vi "Main.vi"(8 "error in (no error)":errorcluster) -> ()   [LabVIEW 2014, in "PmuImpairModule.lvlib"]
uses:
  PmuImpairModule.lvlib
  <userlib>/NIST/ModuleAdminLib/ModuleAdmin/ModuleAdmin.lvclass
  PublicAPI/Arguments/Requests/clStopArgument.ctl
  PmuImpairPlugins/PmuImpairPluginBase_class/PmuImpairPluginBase.lvclass
  <userlib>/NIST/ModuleAdminLib/ModuleAdmin/ModuleAdmin.lvclass/ModuleAdmin.ctl
  <userlib>/NIST/BaseClasses/BasePlugin_class/BasePlugin.lvclass/BasePlugin.ctl
  PmuImpairPlugins/PmuImpairPluginBase_class/TypeDefs/clImpairConfig.ctl
  PmuImpairPlugins/PmuImpairPluginBase_class/PmuImpairPluginBase.lvclass/PmuImpairPluginBase.ctl
  PublicAPI/Arguments/Requests/dblImpairParams.ctl
  EventPlugins/EventPluginBaseClass/TypeDefs/clEvtReportArray.ctl
  EventPlugins/EventPluginBaseClass/TypeDefs/clEvtReport.ctl
  EventPlugins/EventPluginBaseClass/TypeDefs/dblEvtSignalArray.ctl
  EventPlugins/EventPluginBaseClass/TypeDefs/clEvtConfig.ctl
  <vilib>/Utility/error.llb/DialogType.ctl
  <userlib>/NIST/ModuleAdminLib/ModuleAdmin/Accessors/Read ShowPanel_.vi
  <userlib>/NIST/ModuleAdminLib/ModuleAdmin/Accessors/Write ShowPanel_.vi
  <userlib>/NIST/BaseClasses/BasePlugin_class/Accessors/Write PluginIniFilePath.vi
  <userlib>/NIST/BaseClasses/BasePlugin_class/Accessors/Read PluginIniFilePath.vi
  PmuImpairPlugins/PmuImpairPluginBase_class/Accessors/Write BusNumber.vi
  PmuImpairPlugins/PmuImpairPluginBase_class/Accessors/Read BusNumber.vi
  PmuImpairPlugins/PmuImpairPluginBase_class/Accessors/Write dblEventSignalArray.vi
  PmuImpairPlugins/PmuImpairPluginBase_class/Accessors/Write dblEventParams.vi
  PmuImpairPlugins/PmuImpairPluginBase_class/Accessors/Write clEvtConfig.vi
  <userlib>/NIST/ModuleAdminLib/ModuleAdmin/Accessors/Read CloneRegRef.vi
  <vilib>/Utility/error.llb/Error Cluster From Error Code.vi
  PmuImpairPlugins/PmuImpairPluginBase_class/Accessors/Write clImpairConfig.vi
  PmuImpairPlugins/PmuImpairPluginBase_class/Accessors/Read clImpairConfig.vi
  PmuImpairPlugins/PmuImpairPluginBase_class/Accessors/Write dblImpairParams.vi
  PmuImpairPlugins/PmuImpairPluginBase_class/Accessors/Read dblImpairParams.vi
  PmuImpairPlugins/PmuImpairPluginBase_class/Accessors/Get ImpairReports.vi
  <vilib>/ErrorRing/Error Ring.xnode
  <userlib>/NIST/ModuleAdminLib/CloneRegistration/CloneRegistration.lvclass
  <userlib>/NIST/ModuleAdminLib/ModuleAdmin.lvlib
  <userlib>/NIST/BaseClasses/Object_class/BaseObject.lvclass
  EventPlugins/EventPluginBaseClass/EventPluginBaseClass.lvclass
panel:
  out "error out":errorcluster
  in  "ModuleAdmin":refnum<class "ModuleAdmin.lvclass">
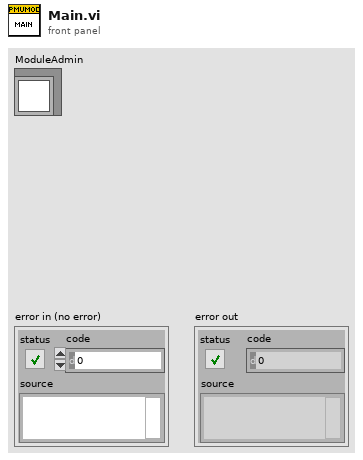
[diagram p1: front panel]
types:
  T1 = typedef "PmuImpairModule.lvlib/clRequestEvents.ctl" = cluster{"StopRequest":refnum<user-event>, "LoadPluginRequest":refnum<user-event>, "WriteImpairConfig":refnum<user-event>, "ReadImpairConfig":refnum<user-event>, "WriteImpairParams":refnum<user-event>, "ReadImpairParams":refnum<user-event>, "WriteEvtReports":refnum<user-event>, "GetImpairReports":refnum<user-event>, "ReadPathToPluginRequest":refnum<user-event>, "WriteEvtSignal":refnum<user-event>, "WriteEvtConfig":refnum<user-event>, "WriteEvtParams":refnum<user-event>, "ReadBusNumber":refnum<user-event>, "WriteBusNumber":refnum<user-event>, "ShowPanel":refnum<user-event>}
  T2 = typedef "PmuImpairModule.lvlib/clBroadcastEvents.ctl" = cluster{"DidInit":refnum<user-event>, "StatusUpdate":refnum<user-event>, "ErrorReport":refnum<user-event>, "DidStop":refnum<user-event>, "ImpairConfig":refnum<user-event>, "ImpairParams":refnum<user-event>, "ImpairReports":refnum<user-event>, "PathToPlugin":refnum<user-event>, "BusNumber":refnum<user-event>}
  T3 = typedef "PmuImpairModule.lvlib/clStopArgument.ctl" = cluster{"Exit via Stop Module Req?":bool, "Wait for Module to stop?":bool, "ModuleAdmin":refnum<class "ModuleAdmin.lvclass">}
  T4 = enum32{"Invalid", "Standard", "Closed", "Hidden", "Minimized", "Maximized"}
  T5 = typedef "PmuImpairPlugins.lvlib/PmuImpairPluginBase.lvclass/clImpairConfig.ctl" = cluster{"FilterType":string, "bPosSeq":bool}
  T6 = typedef "PmuImpairModule.lvlib/dblImpairParams.ctl" = dbl[][]
  T7 = typedef "EventPlugins.lvlib/EventPluginBaseClass.lvclass/clEvtReportArray.ctl" = T8[]
  T8 = typedef "EventPlugins.lvlib/EventPluginBaseClass.lvclass/clEvtReport.ctl" = cluster{"Timestamp":dbl, "Synx":cdb[], "Freq":dbl, "ROCOF":dbl, "ID":i16}
  T9 = typedef "EventPlugins.lvlib/EventPluginBaseClass.lvclass/dblEvtSignalArray.ctl" = dbl[][]
  T10 = typedef "EventPlugins.lvlib/EventPluginBaseClass.lvclass/clEvtConfig.ctl" = cluster{"T0(UTC)":dbl, "F0":dbl, "Fs":i32, "FSamp":u32, "bPosSeq":bool}
  T11 = typedef "DialogType.ctl" = u16
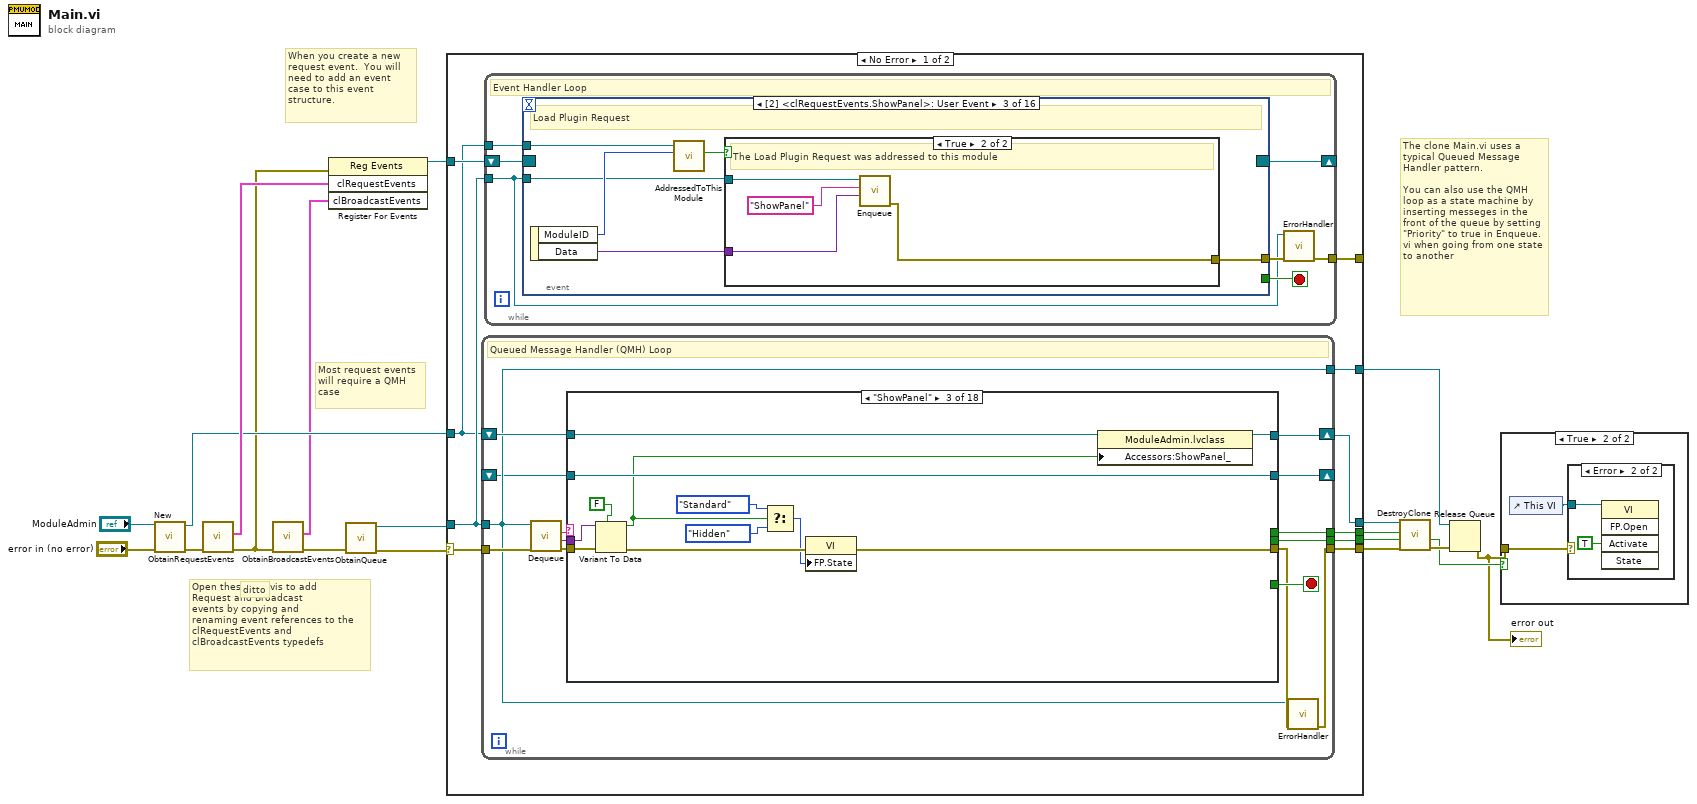
[diagram p0: block diagram]
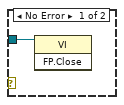
[diagram p3: hidden frame]
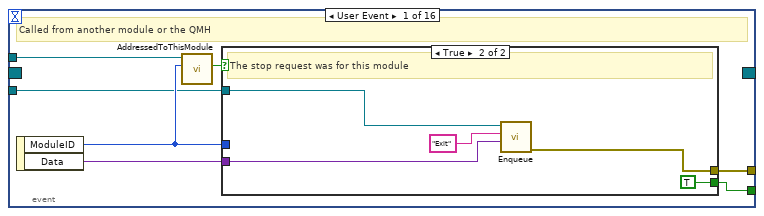
[diagram p4: hidden frame]
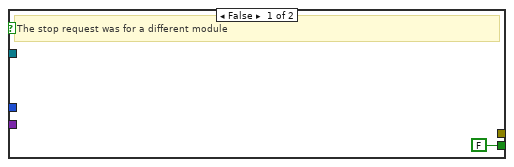
[diagram p5: hidden frame]
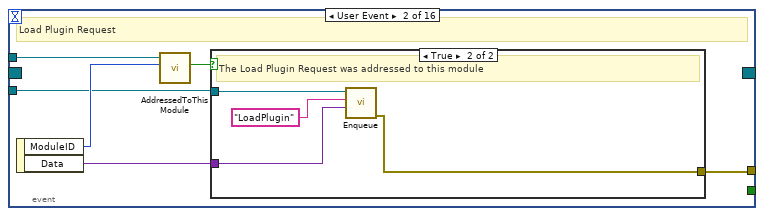
[diagram p6: hidden frame]
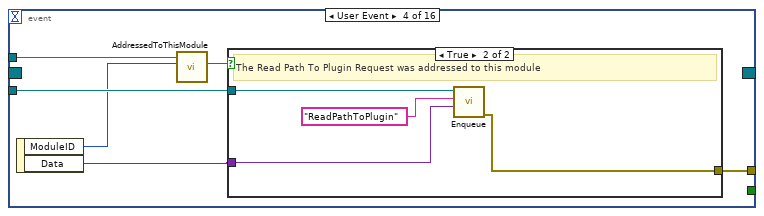
[diagram p9: hidden frame]
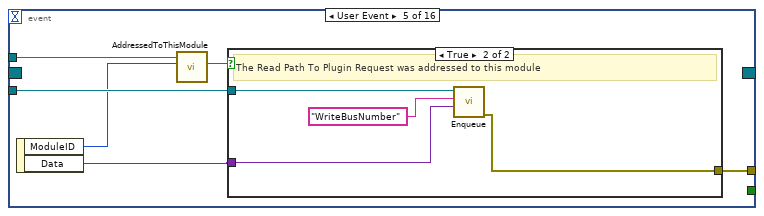
[diagram p11: hidden frame]
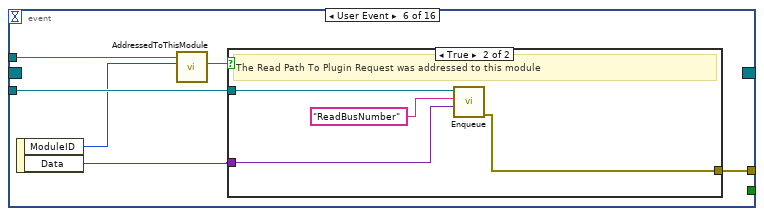
[diagram p13: hidden frame]
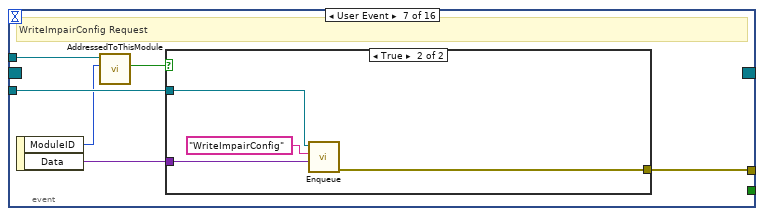
[diagram p15: hidden frame]
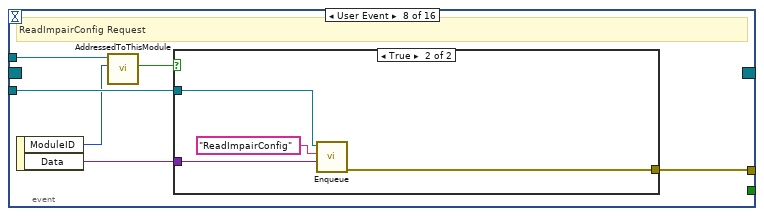
[diagram p17: hidden frame]
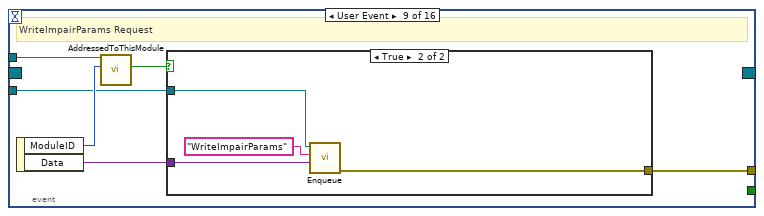
[diagram p19: hidden frame]
diagram:
  # "The clone Main.vi uses a typical Queued Message Handler pattern.  \n\nYou can also use the QMH loop as a state machine by inserting messeges in the front of the queue by setting \"Priority\" to true in Enqueue.vi when going from one state to another"
  # "Open these two vis to add\nRequest and Broadcast \nevents by copying and \nrenaming event references to the \nclRequestEvents and \nclBroadcastEvents typedefs"
  # "ditto"
  # "Most request events\nwill require a QMH\ncase"
  # "When you create a new request event.  You will need to add an event case to this event structure."
  n1 = call <userlib>:"New.vi"("error in (no error)"="error in (no error)", "ModuleAdmin"="ModuleAdmin") -> ("error out"=w17:errorcluster, "ModuleAdmin"=w13:refnum<class "ModuleAdmin.lvclass">)  [unwired: 7 in, 1 out]
  n2 = call "ObtainRequestEvents.vi"("error in (no error)"=w17) -> ("error out"=w10:errorcluster, "clRequestEvents"=w16:T1)  [unwired: 9 in]
  n3 = call "ObtainBroadcastEvents.vi"("error in (no error)"=w10) -> ("error out"=w11:errorcluster, "clBroadcastEvents"=w9:T2)  [unwired: 9 in]
  n4 = register-events(error in=w10, w16, w9) -> (reference out=w8:refnum<event-registration>)  [unwired: 1 in, 1 out]
  n5 = call "ObtainQueue.vi"("error in (no error)"=w11) -> ("error out"=w15:errorcluster, "MessageQueue"=w14:refnum<queue>)  [unwired: 9 in]
  n6 = case shown="No Error" w15 {
    selector: w15 -> [w29 w500]
    tunnel: w14 -> [w27 w496]
    tunnel: w13 -> [w24 w497]
    tunnel: [w28 w498] -> w7
    tunnel: [w26 w496] -> w12
    tunnel: w8 -> [w25 _]
    tunnel: [w23 w495] -> w5
    tunnel: [w22 _] -> w4
    tunnel: [w21 _] -> w3
    tunnel: [w20 _] -> _
    frame No Error {
      n7 = while {
        tunnel: w27 -> [w206]
        tunnel: w29 -> [w215]
        tunnel: [w208] -> w28
        tunnel: [w206] -> w26
        tunnel: [w210] -> w22
        tunnel: [w209] -> w21
        shift-right: [w205] -> _
        shift-left: _ -> [w204]
        shift-right: [w203] -> w23
        shift-left: w24 -> [w211]
        stop <- w216 stop-if-true
        # "Queued Message Handler (QMH) Loop"
        n8 = call "Dequeue.vi"("error in (no error)"=w215, "MessageQueue"=w206) -> ("error out"=w214:errorcluster, "Message Data"=w212:variant, "Message"=w213:string)  [unwired: 6 in, 1 out]
        n9 = case shown="\"ShowPanel\"" w213 {
          selector: w213 -> [w221 _ _ _ _ _ _ _ _ _ _ _ _ _ _ _ _ _]
          tunnel: [_ _ _ _ _ _ _ _ _ _ _ _ _ _ _ _ TRUE _] -> w216
          tunnel: w211 -> [w224 w253 w265 w281 w323 w337 w351 w364 w375 w384 w397 w403 w416 w429 w442 w463 w465 w486]
          tunnel: [w220 w242 w267 w280 w321 w336 w350 w357 w366 w385 w392 w407 w420 w433 w446 w455 w472 w477] -> w207
          tunnel: w214 -> [_ _ w273 w283 w325 w339 w352 w362 w373 w383 w398 w405 w418 w431 w444 w457 w471 w485]
          tunnel: w212 -> [_ _ w272 w284 _ w340 w353 _ _ w382 _ w406 w419 w432 w445 _ w470 w484]
          tunnel: [_ _ _ _ _ _ _ _ _ _ _ _ _ _ _ _ w468 _] -> w210
          tunnel: [_ _ _ _ _ _ _ _ _ _ _ _ _ _ _ _ w467 _] -> w209
          tunnel: [w218 refnum<class "PmuImpairPluginBase.lvclass"> refnum ("PmuImpairPlugins.lvlib:PmuImpairPluginBase.lvclass") w266 w276 w322 w331 w345 w360 w371 w379 w394 w401 w414 w427 w440 w462 w466 w476] -> w205
          tunnel: w204 -> [w218 _ w266 w282 w324 w332 w346 w363 w374 w380 w399 w402 w415 w428 w441 w460 w466 w476]
          tunnel: [w217 w233 w263 w274 w319 w328 w341 w354 w365 w376 w389 w400 w413 w426 w439 w452 w465 w474] -> w203
          frame Default {
            # "Called only if a message was queued and no QMH case was created"
            n10 = property class="ModuleAdmin.lvclass"(reference=w224) -> (reference out=w217:refnum<class "ModuleAdmin.lvclass">, "Accessors:Module ID"=w223:i32, "Accessors:ModuleName"=w219:string)  [unwired: 1 in, 1 out]
            n11 = call <userlib>:"ModuleName.vi"("Name"=w219, "ModuleID"=w223) -> ("ModuleName"=w222:string)  [unwired: 9 in]
            n12 = xnode "Error Ring"("parameter 0"=w221, "parameter 1"=w222) -> ("error out"=w220:errorcluster)
          }
          frame "Initialize" {
            # "Initialize is always called after ObtainQueue.vi is run"
            n13 = property class="ModuleAdmin.lvclass"(reference=w253) -> (reference out=w238:refnum<class "ModuleAdmin.lvclass">, error out=w250:errorcluster, "Accessors:Module ID"=w241:i32, "Accessors:ShowPanel_"=w236:bool, "Accessors:External Launch"=w235:bool, "Accessors:ModuleName"=w237:string)  [unwired: 1 in]
            n14 = Compound Arithmetic op=OR(w236, invert w235) -> (w234:bool)
            n15 = Select(t=T4."Standard" ("Front Panel Window:State"), s=w234, f=T4."Hidden" ("Front Panel Window:State")) -> (s? t:f=w246:T4)
            n16 = invoke class="VI" method="FP.Open"(error in=w250, "State"=w246) -> (error out=w249:errorcluster)  [unwired: 3 in, 4 out]
            n17 = call <userlib>:"ModuleName.vi"("Name"=w237, "ModuleID"=w241) -> ("ModuleName"=w245:string)  [unwired: 9 in]
            n18 = property class="VI"(error in=w249, "Front Panel.Title"=w245) -> (reference out=w252:refnum<vi>, error out=w251:errorcluster)  [unwired: 1 in]
            n19 = invoke class="VI" method="FP.Center"(reference=w252, error in=w251) -> (error out=w240:errorcluster)  [unwired: 1 in, 2 out]
            n20 = case shown="True" w235 {
              tunnel: [w254 w260] -> w243
              tunnel: [w255 w257] -> w233
              tunnel: w240 -> [w254 w259]
              tunnel: w238 -> [w255 w256]
              frame False {
              }
              frame True {
                n21 = call <userlib>:"WaitOnModuleSync.vi"("error in (no error)"=w259, "ModuleAdmin"=w256) -> ("error out"=w261:errorcluster, "ModuleAdmin"=w258:refnum<class "ModuleAdmin.lvclass">)  [unwired: 8 in]
                n22 = call <userlib>:"WaitOnEventSync.vi"("error in (no error)"=w261, "ModuleAdmin"=w258) -> ("error out"=w260:errorcluster, "ModuleAdmin"=w257:refnum<class "ModuleAdmin.lvclass">)  [unwired: 8 in]
              }
            }
            n23 = call "DidInit.vi"("Init?"=TRUE, "error in (no error)"=w243, "ModuleAdmin"=w233) -> ("error out"=w242:errorcluster)  [unwired: 8 in]
          }
          frame "ShowPanel" {
            n24 = Variant To Data(error in=w273, type=FALSE, Variant=w272) -> (data=w264:bool, error out=w269:errorcluster)
            n25 = Select(t=T4."Standard" ("Front Panel Window:State"), s=w264, f=T4."Hidden" ("Front Panel Window:State")) -> (s? t:f=w268:T4)
            n26 = property class="VI"(error in=w269, "FP.State"=w268) -> (error out=w267:errorcluster)  [unwired: 1 in, 1 out]
            n27 = property class="ModuleAdmin.lvclass"(reference=w265, "Accessors:ShowPanel_"=w264) -> (reference out=w263:refnum<class "ModuleAdmin.lvclass">)  [unwired: 1 in, 1 out]
          }
          frame "LoadPlugin" {
            # "Load plugin from ImpairPlugins and broadcast status update."
            n28 = Variant To Data(error in=w283, type=path "", Variant=w284) -> (data=w275:path, error out=w289:errorcluster)
            n29 = call <userlib>:"GetPathToClass.vi"("error in (no error)"=w289, "configuration file path"=w275) -> ("error IO"=w288:errorcluster, "PathToClass"=w278:path)  [unwired: 8 in]
            n30 = Current VI's Path() -> (path=w279:path)
            n31 = Build Path(base path=w279, name or relative path=w278) -> (appended path=w277:path)
            n32 = call <vilib>:"Check if File or Folder Exists.vi"("error in (no error)"=w288, "path"=w277) -> ("error out"=w286:errorcluster, "file or folder exists?"=w287:bool, "dup path"=w285:path)  [unwired: 7 in]
            n33 = case shown="True" w287 {
              tunnel: w285 -> [w295 w310]
              tunnel: w286 -> [w296 w307]
              tunnel: [w301 w308] -> w280
              tunnel: w282 -> [_ w306]
              tunnel: w281 -> [w298 w305]
              tunnel: [w293 w306] -> w276
              tunnel: w275 -> [w292 _]
              tunnel: [w291 w305] -> w274
              frame True {
                n34 = property class="ModuleAdmin.lvclass"(reference=w298) -> (reference out=w291:refnum<class "ModuleAdmin.lvclass">, "Accessors:Module ID"=w299:i32)  [unwired: 1 in, 1 out]
                n35 = call-dynamic "LoadClassFromFile.vi"("error in (no error)"=w296, "class path"=w295, "reference in"=refnum<class "PmuImpairPluginBase.lvclass"> refnum ("PmuImpairPlugins.lvlib:PmuImpairPluginBase.lvclass")) -> ("error out"=w300:errorcluster, "reference out"=w294:refnum<class "PmuImpairPluginBase.lvclass">)  [unwired: 7 in]
                n36 = property class="PmuImpairPluginBase.lvclass"(reference=w294, "Accessors:PluginIniFilePath"=w292) -> (reference out=w293:refnum<class "PmuImpairPluginBase.lvclass">)  [unwired: 1 in, 1 out]
                n37 = Path To String(path=w295) -> (string=w303:string)
                n38 = Format Into String(format string="Plugin %s  loaded", w303) -> (resulting string=w302:string)  [unwired: 2 in, 1 out]
                n39 = call "StatusUpdate.vi"("error in (no error)"=w300, "Status"=w302, "ModuleID"=w299) -> ("error out"=w301:errorcluster)  [unwired: 8 in]
              }
              frame False {
                n40 = Path To String(path=w310) -> (string=w309:string)
                n41 = xnode "Error Ring"("parameter 0"=w309) -> ("error out"=w311:errorcluster)
                n42 = Merge Errors(w311, w307) -> (w308:errorcluster)
              }
            }
          }
          frame "ReadPathToPlugin" {
            # "Read the PmuImpairPluginINIFilePath and broadcast this path as part of the Load Plugin cluster."
            n43 = property class="PmuImpairPluginBase.lvclass"(reference=w324, error in=w325) -> (reference out=w322:refnum<class "PmuImpairPluginBase.lvclass">, error out=w326:errorcluster, "Accessors:PluginIniFilePath"=w320:path)
            n44 = property class="ModuleAdmin.lvclass"(reference=w323) -> (reference out=w319:refnum<class "ModuleAdmin.lvclass">, "Accessors:Module ID"=w327:i32)  [unwired: 1 in, 1 out]
            n45 = call "ReadPathToPlugin.vi"("error in (no error)"=w326, "PmuImpairPluginINIFilePath"=w320, "ModuleID"=w327) -> ("error out"=w321:errorcluster)  [unwired: 8 in]
          }
          frame "WriteImpairConfig" {
            # "Write Impairment Configuration (cluster) and broadcast status update."
            n46 = Variant To Data(error in=w339, type=T5 {"FilterType"="", "bPosSeq"=TRUE} ("clImpairConfig"), Variant=w340) -> (data=w329:T5, error out=w330:errorcluster)
            n47 = property class="PmuImpairPluginBase.lvclass"(reference=w332, error in=w330, "Accessors:clImpairConfig"=w329) -> (reference out=w331:refnum<class "PmuImpairPluginBase.lvclass">, error out=w333:errorcluster)
            n48 = property class="ModuleAdmin.lvclass"(reference=w337) -> (reference out=w328:refnum<class "ModuleAdmin.lvclass">, "Accessors:Module ID"=w335:i32)  [unwired: 1 in, 1 out]
            n49 = call "StatusUpdate.vi"("error in (no error)"=w333, "Status"="Config Received", "ModuleID"=w335) -> ("error out"=w336:errorcluster)  [unwired: 8 in]
          }
          frame "WriteBusNumber" {
            # "Write Impairment Configuration (cluster) and broadcast status update."
            n50 = Variant To Data(error in=w352, type=u8 0 ("BusNumber"), Variant=w353) -> (data=w342:u8, error out=w344:errorcluster)
            n51 = property class="PmuImpairPluginBase.lvclass"(reference=w346, error in=w344, "Accessors:BusNumber"=w342) -> (reference out=w345:refnum<class "PmuImpairPluginBase.lvclass">, error out=w347:errorcluster)
            n52 = property class="ModuleAdmin.lvclass"(reference=w351) -> (reference out=w341:refnum<class "ModuleAdmin.lvclass">, "Accessors:Module ID"=w349:i32)  [unwired: 1 in, 1 out]
            n53 = call "StatusUpdate.vi"("error in (no error)"=w347, "Status"="Bus Number Received", "ModuleID"=w349) -> ("error out"=w350:errorcluster)  [unwired: 8 in]
          }
          frame "ReadImpairConfig" {
            # "Read Impairment Configuration (cluster) and broadcast a user event to display the values in the API."
            n54 = property class="PmuImpairPluginBase.lvclass"(reference=w363, error in=w362) -> (reference out=w360:refnum<class "PmuImpairPluginBase.lvclass">, error out=w361:errorcluster, "Accessors:clImpairConfig"=w359:T5)
            n55 = property class="ModuleAdmin.lvclass"(reference=w364) -> (reference out=w354:refnum<class "ModuleAdmin.lvclass">, "Accessors:Module ID"=w356:i32)  [unwired: 1 in, 1 out]
            n56 = call "ReadImpairConfig.vi"("error in (no error)"=w361, "clImpairConfigReport"=w359, "ModuleID"=w356) -> ("error out"=w358:errorcluster)  [unwired: 8 in]
            n57 = call "StatusUpdate.vi"("error in (no error)"=w358, "Status"="Config Transmitted", "ModuleID"=w356) -> ("error out"=w357:errorcluster)  [unwired: 8 in]
          }
          frame "ReadBusNumber" {
            # "Read Impairment Configuration (cluster) and broadcast a user event to display the values in the API."
            n58 = property class="PmuImpairPluginBase.lvclass"(reference=w374, error in=w373) -> (reference out=w371:refnum<class "PmuImpairPluginBase.lvclass">, error out=w372:errorcluster, "Accessors:BusNumber"=w370:u8)
            n59 = property class="ModuleAdmin.lvclass"(reference=w375) -> (reference out=w365:refnum<class "ModuleAdmin.lvclass">, "Accessors:Module ID"=w368:i32)  [unwired: 1 in, 1 out]
            n60 = call "ReadBusNumber.vi"("error in (no error)"=w372, "BusNumber"=w370, "ModuleID"=w368) -> ("error out"=w369:errorcluster)  [unwired: 8 in]
            n61 = call "StatusUpdate.vi"("error in (no error)"=w369, "Status"="BusNumber Transmitted", "ModuleID"=w368) -> ("error out"=w366:errorcluster)  [unwired: 8 in]
          }
          frame "WriteImpairParams" {
            w381 = T6 []  # dblImpairParams
            # "Write Impairment Parameters (2-d array) and broadcast status update."
            n62 = Variant To Data(error in=w383, type=w381, Variant=w382) -> (data=w377:T6, error out=w378:errorcluster)
            n63 = property class="PmuImpairPluginBase.lvclass"(reference=w380, error in=w378, "Accessors:dblImpairParams"=w377) -> (reference out=w379:refnum<class "PmuImpairPluginBase.lvclass">, error out=w386:errorcluster)
            n64 = property class="ModuleAdmin.lvclass"(reference=w384) -> (reference out=w376:refnum<class "ModuleAdmin.lvclass">, "Accessors:Module ID"=w388:i32)  [unwired: 1 in, 1 out]
            n65 = call "StatusUpdate.vi"("error in (no error)"=w386, "Status"="Params Received", "ModuleID"=w388) -> ("error out"=w385:errorcluster)  [unwired: 8 in]
          }
          frame "ReadImpairParams" {
            # "Read Impairment Parameters (2-d array) and broadcast a user event to display the values in the API."
            n66 = property class="PmuImpairPluginBase.lvclass"(reference=w399, error in=w398) -> (reference out=w394:refnum<class "PmuImpairPluginBase.lvclass">, error out=w395:errorcluster, "Accessors:dblImpairParams"=w396:dbl[][])
            n67 = property class="ModuleAdmin.lvclass"(reference=w397) -> (reference out=w389:refnum<class "ModuleAdmin.lvclass">, "Accessors:Module ID"=w390:i32)  [unwired: 1 in, 1 out]
            n68 = call "ReadImpairParams.vi"("error in (no error)"=w395, "clImpairParamsReport"=w396, "ModuleID"=w390) -> ("error out"=w393:errorcluster)  [unwired: 8 in]
            n69 = call "StatusUpdate.vi"("error in (no error)"=w393, "Status"="Params Transmitted", "ModuleID"=w390) -> ("error out"=w392:errorcluster)  [unwired: 8 in]
          }
          frame "WriteEvtReports" {
            w404 = T7 []  # EvtReportArray
            # "Write Event Reports (array of clusters) and broadcast status update."
            n70 = Variant To Data(error in=w405, type=w404, Variant=w406) -> (data=w408:T7, error out=w409:errorcluster)
            n71 = property class="PmuImpairPluginBase.lvclass"(reference=w402, error in=w409, "Accessors:clEvtReportArray"=w408) -> (reference out=w401:refnum<class "PmuImpairPluginBase.lvclass">, error out=w410:errorcluster)
            n72 = property class="ModuleAdmin.lvclass"(reference=w403) -> (reference out=w400:refnum<class "ModuleAdmin.lvclass">, "Accessors:Module ID"=w412:i32)  [unwired: 1 in, 1 out]
            n73 = call "StatusUpdate.vi"("error in (no error)"=w410, "Status"="Event Reports Received", "ModuleID"=w412) -> ("error out"=w407:errorcluster)  [unwired: 8 in]
          }
          frame "WriteEvtSignal" {
            w417 = T9 []  # EvtSignal
            # "Write Event Signal and broadcast status update."
            n74 = Variant To Data(error in=w418, type=w417, Variant=w419) -> (data=w421:T9, error out=w422:errorcluster)
            n75 = property class="PmuImpairPluginBase.lvclass"(reference=w415, error in=w422, "Accessors:dblEventSignalArray"=w421) -> (reference out=w414:refnum<class "PmuImpairPluginBase.lvclass">, error out=w423:errorcluster)
            n76 = property class="ModuleAdmin.lvclass"(reference=w416) -> (reference out=w413:refnum<class "ModuleAdmin.lvclass">, "Accessors:Module ID"=w425:i32)  [unwired: 1 in, 1 out]
            n77 = call "StatusUpdate.vi"("error in (no error)"=w423, "Status"="Event Signal Received", "ModuleID"=w425) -> ("error out"=w420:errorcluster)  [unwired: 8 in]
          }
          frame "WriteEvtParams" {
            w430 = T9 []  # EvtParams
            # "Write Event Signal and broadcast status update."
            n78 = Variant To Data(error in=w431, type=w430, Variant=w432) -> (data=w434:T9, error out=w435:errorcluster)
            n79 = property class="PmuImpairPluginBase.lvclass"(reference=w428, error in=w435, "Accessors:dblEventParams"=w434) -> (reference out=w427:refnum<class "PmuImpairPluginBase.lvclass">, error out=w436:errorcluster)
            n80 = property class="ModuleAdmin.lvclass"(reference=w429) -> (reference out=w426:refnum<class "ModuleAdmin.lvclass">, "Accessors:Module ID"=w438:i32)  [unwired: 1 in, 1 out]
            n81 = call "StatusUpdate.vi"("error in (no error)"=w436, "Status"="Event Params Received", "ModuleID"=w438) -> ("error out"=w433:errorcluster)  [unwired: 8 in]
          }
          frame "WriteEvtConfig" {
            w443 = T10 {"T0(UTC)"=0.0, "F0"=0.0, "Fs"=0, "FSamp"=0, "bPosSeq"=FALSE}  # EvtConfig
            # "Write Event Signal and broadcast status update."
            n82 = Variant To Data(error in=w444, type=w443, Variant=w445) -> (data=w447:T10, error out=w448:errorcluster)
            n83 = property class="PmuImpairPluginBase.lvclass"(reference=w441, error in=w448, "Accessors:clEvtConfig"=w447) -> (reference out=w440:refnum<class "PmuImpairPluginBase.lvclass">, error out=w449:errorcluster)
            n84 = property class="ModuleAdmin.lvclass"(reference=w442) -> (reference out=w439:refnum<class "ModuleAdmin.lvclass">, "Accessors:Module ID"=w451:i32)  [unwired: 1 in, 1 out]
            n85 = call "StatusUpdate.vi"("error in (no error)"=w449, "Status"="Event Config Received", "ModuleID"=w451) -> ("error out"=w446:errorcluster)  [unwired: 8 in]
          }
          frame "GetImpairReports" {
            n86 = call-dynamic "GetImpairReports.vi"("error in (no error)"=w457, "PmuImpairPluginBase in"=w460) -> ("error out"=w458:errorcluster, "PmuImpairPluginBase out"=w459:refnum<class "PmuImpairPluginBase.lvclass">)  [unwired: 8 in]
            n87 = property class="PmuImpairPluginBase.lvclass"(reference=w459, error in=w458) -> (reference out=w462:refnum<class "PmuImpairPluginBase.lvclass">, error out=w464:errorcluster, "Accessors:clImpairReportArray"=w461:T7)
            n88 = property class="ModuleAdmin.lvclass"(reference=w463) -> (reference out=w452:refnum<class "ModuleAdmin.lvclass">, "Accessors:Module ID"=w454:i32)  [unwired: 1 in, 1 out]
            n89 = call "GetImpairReports.vi"("error in (no error)"=w464, "clPmuImpairRptArray"=w461, "ModuleID"=w454) -> ("error out"=w456:errorcluster)  [unwired: 8 in]
            n90 = call "StatusUpdate.vi"("error in (no error)"=w456, "Status"="Impairment Reports Transmitted", "ModuleID"=w454) -> ("error out"=w455:errorcluster)  [unwired: 8 in]
          }
          frame "Exit" {
            # "Called by the StopRequest event handler case"
            n91 = control-ref of="This VI"() -> (w469:refnum<vi>)
            n92 = call "HandleExit.vi"("error in (no error)"=w471, "VI Refnum"=w469, "StopArgument"=w470, "ModuleAdmin"=w465) -> ("error out"=w472:errorcluster, "Exit via Stop Module Req?"=w467:bool, "WaitForStop?"=w468:bool)  [unwired: 5 in]
          }
          frame "Error" {
            n93 = property class="ModuleAdmin.lvclass"(reference=w486) -> (reference out=w475:refnum<class "ModuleAdmin.lvclass">, "Accessors:External Launch"=w480:bool, "Accessors:Module ID"=w478:i32)  [unwired: 1 in, 1 out]
            n94 = Variant To Data(error in=w485, type=errorcluster {"status"=FALSE, "code"=0, "source"=""} ("error constant"), Variant=w484) -> (data=w479:errorcluster, error out=w482:errorcluster)
            n95 = call "ReportError.vi"("error in (no error)"=w482, "ErrorReported"=w479, "ModuleID"=w478) -> ("error out"=w481:errorcluster)  [unwired: 8 in]
            n96 = case shown="True" w480 {
              tunnel: w481 -> [w490 w492]
              tunnel: w479 -> [w489 _]
              tunnel: [w488 w492] -> w477
              tunnel: w475 -> [w487 w491]
              tunnel: [w487 w491] -> w474
              frame False {
                # "Todo:  Add an event to ask the user\nIf the module should stop or continue"
                # "Stand alone: now, force an exit"
                n97 = call <vilib>:"Simple Error Handler.vi"("error in (no error)"=w489) -> ()  [unwired: 4 in, 5 out]
                n98 = call "StopRequest.vi"("error in (no error)"=w490, "ModuleAdmin"=w487) -> ("error out"=w488:errorcluster)  [unwired: 8 in, 1 out]
              }
              frame True {
                # "Externally launched modules only broadcast the error msg"
              }
            }
          }
        }
        n99 = call "ErrorHandler.vi"("error in (no error)"=w207, "MessageQueue"=w206) -> ("error out"=w208:errorcluster)  [unwired: 8 in, 1 out]
      }
      n100 = while {
        tunnel: w27 -> [w30]
        shift-right: [w34] -> _
        shift-left: w25 -> [w35]
        tunnel: w24 -> [w33]
        tunnel: [w31] -> w20
        stop <- w36 stop-if-true
        # "Event Handler Loop"
        n101 = event shown="[2] <clRequestEvents.ShowPanel>: User Event" {
          selector: w35 -> [_ _ _ _ _ _ _ _ _ _ _ _ _ _ _ _]
          dyn-events: [_ _ _ _ _ _ _ _ _ _ _ _ _ _ _ _] -> w34
          timeout: _ -> [_ _ _ _ _ _ _ _ _ _ _ _ _ _ _ _]
          tunnel: w30 -> [w40 w51 w61 w73 w83 w93 w103 w112 w121 w132 w141 w151 w161 w171 w183 w202]
          tunnel: [w39 _ _ _ _ _ _ _ _ _ _ _ _ _ _ TRUE] -> w36
          tunnel: w33 -> [w43 w54 w64 w72 w82 w92 w101 w114 w122 w134 w143 w153 w163 w173 w184 w196]
          tunnel: [w38 w52 w62 w74 w84 w94 w102 w111 w120 w130 w140 w150 w160 w170 w180 w200] -> w32
          event User Event {
            # "Called from another module or the QMH"
            n102 = event-data() -> ("ModuleID"=w41:i32, "Data"=w37:variant)  [unwired: 1 in]
            n103 = call <userlib>:"AddressedToThisModule.vi"("ModuleID"=w41, "ModuleAdmin"=w43) -> ("AddressedToThisInstance?"=w42:bool)  [unwired: 8 in, 1 out]
            n104 = case shown="True" w42 {
              tunnel: w41 -> [_ _]
              tunnel: w40 -> [_ w49]
              tunnel: [FALSE TRUE] -> w39
              tunnel: [_ w47] -> w38
              tunnel: w37 -> [_ w45]
              frame False {
                # "The stop request was for a different module"
              }
              frame True {
                # "The stop request was for this module"
                n105 = call "Enqueue.vi"("Message Data"=w45, "Message"="Exit", "MessageQueue"=w49) -> ("error out"=w47:errorcluster)  [unwired: 7 in, 1 out]
              }
            }
          }
          event User Event {
            # "Load Plugin Request"
            n106 = event-data() -> ("ModuleID"=w53:i32, "Data"=w50:variant)  [unwired: 1 in]
            n107 = call <userlib>:"AddressedToThisModule.vi"("ModuleID"=w53, "ModuleAdmin"=w54) -> ("AddressedToThisInstance?"=w55:bool)  [unwired: 8 in, 1 out]
            n108 = case shown="True" w55 {
              tunnel: w50 -> [_ w59]
              tunnel: [_ w57] -> w52
              tunnel: w51 -> [_ w56]
              frame False {
                # "Not addressed to this module"
              }
              frame True {
                # "The Load Plugin Request was addressed to this module"
                n109 = call "Enqueue.vi"("Message Data"=w59, "Message"="LoadPlugin", "MessageQueue"=w56) -> ("error out"=w57:errorcluster)  [unwired: 7 in, 1 out]
              }
            }
          }
          event User Event {
            # "Load Plugin Request"
            n110 = event-data() -> ("ModuleID"=w63:i32, "Data"=w60:variant)  [unwired: 1 in]
            n111 = call <userlib>:"AddressedToThisModule.vi"("ModuleID"=w63, "ModuleAdmin"=w64) -> ("AddressedToThisInstance?"=w65:bool)  [unwired: 8 in, 1 out]
            n112 = case shown="True" w65 {
              tunnel: w60 -> [_ w69]
              tunnel: [_ w67] -> w62
              tunnel: w61 -> [_ w66]
              frame False {
                # "Not addressed to this module"
              }
              frame True {
                # "The Load Plugin Request was addressed to this module"
                n113 = call "Enqueue.vi"("Message Data"=w69, "Message"="ShowPanel", "MessageQueue"=w66) -> ("error out"=w67:errorcluster)  [unwired: 7 in, 1 out]
              }
            }
          }
          event User Event {
            n114 = event-data() -> ("ModuleID"=w71:i32, "Data"=w70:variant)  [unwired: 1 in]
            n115 = call <userlib>:"AddressedToThisModule.vi"("ModuleID"=w71, "ModuleAdmin"=w72) -> ("AddressedToThisInstance?"=w75:bool)  [unwired: 8 in, 1 out]
            n116 = case shown="True" w75 {
              tunnel: w70 -> [_ w79]
              tunnel: [_ w77] -> w74
              tunnel: w73 -> [_ w76]
              frame False {
                # "Not addressed to this module"
              }
              frame True {
                # "The Read Path To Plugin Request was addressed to this module"
                n117 = call "Enqueue.vi"("Message Data"=w79, "Message"="ReadPathToPlugin", "MessageQueue"=w76) -> ("error out"=w77:errorcluster)  [unwired: 7 in, 1 out]
              }
            }
          }
          event User Event {
            n118 = event-data() -> ("ModuleID"=w81:i32, "Data"=w80:variant)  [unwired: 1 in]
            n119 = call <userlib>:"AddressedToThisModule.vi"("ModuleID"=w81, "ModuleAdmin"=w82) -> ("AddressedToThisInstance?"=w85:bool)  [unwired: 8 in, 1 out]
            n120 = case shown="True" w85 {
              tunnel: w80 -> [_ w89]
              tunnel: [_ w87] -> w84
              tunnel: w83 -> [_ w86]
              frame False {
                # "Not addressed to this module"
              }
              frame True {
                # "The Read Path To Plugin Request was addressed to this module"
                n121 = call "Enqueue.vi"("Message Data"=w89, "Message"="WriteBusNumber", "MessageQueue"=w86) -> ("error out"=w87:errorcluster)  [unwired: 7 in, 1 out]
              }
            }
          }
          event User Event {
            n122 = event-data() -> ("ModuleID"=w91:i32, "Data"=w90:variant)  [unwired: 1 in]
            n123 = call <userlib>:"AddressedToThisModule.vi"("ModuleID"=w91, "ModuleAdmin"=w92) -> ("AddressedToThisInstance?"=w95:bool)  [unwired: 8 in, 1 out]
            n124 = case shown="True" w95 {
              tunnel: w90 -> [_ w99]
              tunnel: [_ w97] -> w94
              tunnel: w93 -> [_ w96]
              frame False {
                # "Not addressed to this module"
              }
              frame True {
                # "The Read Path To Plugin Request was addressed to this module"
                n125 = call "Enqueue.vi"("Message Data"=w99, "Message"="ReadBusNumber", "MessageQueue"=w96) -> ("error out"=w97:errorcluster)  [unwired: 7 in, 1 out]
              }
            }
          }
          event User Event {
            # "WriteImpairConfig Request"
            n126 = event-data() -> ("ModuleID"=w100:i32, "Data"=w104:variant)  [unwired: 1 in]
            n127 = call <userlib>:"AddressedToThisModule.vi"("ModuleID"=w100, "ModuleAdmin"=w101) -> ("AddressedToThisInstance?"=w105:bool)  [unwired: 8 in, 1 out]
            n128 = case shown="True" w105 {
              tunnel: [_ w106] -> w102
              tunnel: w104 -> [_ w108]
              tunnel: w103 -> [_ w107]
              frame False {
              }
              frame True {
                n129 = call "Enqueue.vi"("Message Data"=w108, "Message"="WriteImpairConfig", "MessageQueue"=w107) -> ("error out"=w106:errorcluster)  [unwired: 7 in, 1 out]
              }
            }
          }
          event User Event {
            # "ReadImpairConfig Request"
            n130 = event-data() -> ("ModuleID"=w110:i32, "Data"=w113:variant)  [unwired: 1 in]
            n131 = call <userlib>:"AddressedToThisModule.vi"("ModuleID"=w110, "ModuleAdmin"=w114) -> ("AddressedToThisInstance?"=w115:bool)  [unwired: 8 in, 1 out]
            n132 = case shown="True" w115 {
              tunnel: [_ w118] -> w111
              tunnel: w113 -> [_ w117]
              tunnel: w112 -> [_ w116]
              frame False {
              }
              frame True {
                n133 = call "Enqueue.vi"("Message Data"=w117, "Message"="ReadImpairConfig", "MessageQueue"=w116) -> ("error out"=w118:errorcluster)  [unwired: 7 in, 1 out]
              }
            }
          }
          event User Event {
            # "WriteImpairParams Request"
            n134 = event-data() -> ("ModuleID"=w123:i32, "Data"=w124:variant)  [unwired: 1 in]
            n135 = call <userlib>:"AddressedToThisModule.vi"("ModuleID"=w123, "ModuleAdmin"=w122) -> ("AddressedToThisInstance?"=w125:bool)  [unwired: 8 in, 1 out]
            n136 = case shown="True" w125 {
              tunnel: [_ w128] -> w120
              tunnel: w124 -> [_ w127]
              tunnel: w121 -> [_ w126]
              frame False {
              }
              frame True {
                n137 = call "Enqueue.vi"("Message Data"=w127, "Message"="WriteImpairParams", "MessageQueue"=w126) -> ("error out"=w128:errorcluster)  [unwired: 7 in, 1 out]
              }
            }
          }
          event User Event {
            # "ReadImpairParams Request"
            n138 = event-data() -> ("ModuleID"=w133:i32, "Data"=w131:variant)  [unwired: 1 in]
            n139 = call <userlib>:"AddressedToThisModule.vi"("ModuleID"=w133, "ModuleAdmin"=w134) -> ("AddressedToThisInstance?"=w135:bool)  [unwired: 8 in, 1 out]
            n140 = case shown="True" w135 {
              tunnel: [_ w138] -> w130
              tunnel: w132 -> [_ w137]
              tunnel: w131 -> [_ w136]
              frame False {
              }
              frame True {
                n141 = call "Enqueue.vi"("Message Data"=w136, "Message"="ReadImpairParams", "MessageQueue"=w137) -> ("error out"=w138:errorcluster)  [unwired: 7 in, 1 out]
              }
            }
          }
          event User Event {
            # "WriteEvtReports Request"
            n142 = event-data() -> ("ModuleID"=w142:i32, "Data"=w144:variant)  [unwired: 1 in]
            n143 = call <userlib>:"AddressedToThisModule.vi"("ModuleID"=w142, "ModuleAdmin"=w143) -> ("AddressedToThisInstance?"=w145:bool)  [unwired: 8 in, 1 out]
            n144 = case shown="True" w145 {
              tunnel: [_ w148] -> w140
              tunnel: w144 -> [_ w147]
              tunnel: w141 -> [_ w146]
              frame False {
              }
              frame True {
                n145 = call "Enqueue.vi"("Message Data"=w147, "Message"="WriteEvtReports", "MessageQueue"=w146) -> ("error out"=w148:errorcluster)  [unwired: 7 in, 1 out]
              }
            }
          }
          event User Event {
            # "WriteEvtSignal Request"
            n146 = event-data() -> ("ModuleID"=w152:i32, "Data"=w154:variant)  [unwired: 1 in]
            n147 = call <userlib>:"AddressedToThisModule.vi"("ModuleID"=w152, "ModuleAdmin"=w153) -> ("AddressedToThisInstance?"=w155:bool)  [unwired: 8 in, 1 out]
            n148 = case shown="True" w155 {
              tunnel: [_ w158] -> w150
              tunnel: w154 -> [_ w157]
              tunnel: w151 -> [_ w156]
              frame False {
              }
              frame True {
                n149 = call "Enqueue.vi"("Message Data"=w157, "Message"="WriteEvtSignal", "MessageQueue"=w156) -> ("error out"=w158:errorcluster)  [unwired: 7 in, 1 out]
              }
            }
          }
          event User Event {
            # "WriteEvtSignal Request"
            n150 = event-data() -> ("ModuleID"=w162:i32, "Data"=w164:variant)  [unwired: 1 in]
            n151 = call <userlib>:"AddressedToThisModule.vi"("ModuleID"=w162, "ModuleAdmin"=w163) -> ("AddressedToThisInstance?"=w165:bool)  [unwired: 8 in, 1 out]
            n152 = case shown="True" w165 {
              tunnel: [_ w168] -> w160
              tunnel: w164 -> [_ w167]
              tunnel: w161 -> [_ w166]
              frame False {
              }
              frame True {
                n153 = call "Enqueue.vi"("Message Data"=w167, "Message"="WriteEvtParams", "MessageQueue"=w166) -> ("error out"=w168:errorcluster)  [unwired: 7 in, 1 out]
              }
            }
          }
          event User Event {
            # "WriteEvtSignal Request"
            n154 = event-data() -> ("ModuleID"=w172:i32, "Data"=w174:variant)  [unwired: 1 in]
            n155 = call <userlib>:"AddressedToThisModule.vi"("ModuleID"=w172, "ModuleAdmin"=w173) -> ("AddressedToThisInstance?"=w175:bool)  [unwired: 8 in, 1 out]
            n156 = case shown="True" w175 {
              tunnel: [_ w178] -> w170
              tunnel: w174 -> [_ w177]
              tunnel: w171 -> [_ w176]
              frame False {
              }
              frame True {
                n157 = call "Enqueue.vi"("Message Data"=w177, "Message"="WriteEvtConfig", "MessageQueue"=w176) -> ("error out"=w178:errorcluster)  [unwired: 7 in, 1 out]
              }
            }
          }
          event User Event {
            # "GetImpairReports Request"
            n158 = event-data() -> ("ModuleID"=w181:i32, "Data"=w182:variant)  [unwired: 1 in]
            n159 = call <userlib>:"AddressedToThisModule.vi"("ModuleID"=w181, "ModuleAdmin"=w184) -> ("AddressedToThisInstance?"=w185:bool)  [unwired: 8 in, 1 out]
            n160 = case shown="True" w185 {
              tunnel: [_ w188] -> w180
              tunnel: w183 -> [_ w187]
              tunnel: w182 -> [_ w186]
              frame False {
              }
              frame True {
                n161 = call "Enqueue.vi"("Message Data"=w186, "Message"="GetImpairReports", "MessageQueue"=w187) -> ("error out"=w188:errorcluster)  [unwired: 7 in, 1 out]
              }
            }
          }
          event Panel Close? {
            # "Hide on external launch"
            # "Discard the event so the QMH can complete"
            # "Called from another module or the QMH"
            n162 = event-data() -> ()  [unwired: 1 in, 1 out]
            n163 = property class="ModuleAdmin.lvclass"(reference=w196) -> ("Accessors:External Launch"=w191:bool)  [unwired: 1 in, 2 out]
            n164 = Bundle By Name(cluster=T3 {"Exit via Stop Module Req?"=FALSE, "Wait for Module to stop?"=FALSE, "ModuleAdmin"=refnum} ("Stop Argument"), "Wait for Module to stop?"=FALSE, "Exit via Stop Module Req?"=TRUE) -> (w197:T3)
            n165 = Select(t="HidePanel", s=w191, f="Exit" ("Message")) -> (s? t:f=w193:string)
            n166 = call "Enqueue.vi"("Message Data"=w197, "Message"=w193, "MessageQueue"=w202) -> ("error out"=w200:errorcluster)  [unwired: 7 in, 1 out]
            n167 = event-data("Discard?"=TRUE) -> ()  [unwired: 1 in, 1 out]
          }
        }
        n168 = call "ErrorHandler.vi"("error in (no error)"=w32, "MessageQueue"=w30) -> ("error out"=w31:errorcluster)  [unwired: 8 in, 1 out]
      }
    }
    frame Error {
      n169 = property class="ModuleAdmin.lvclass"(reference=w497) -> (reference out=w495:refnum<class "ModuleAdmin.lvclass">, "Accessors:CloneRegRef"=w494:refnum<data-value>, "Accessors:Module ID"=w493:i32)  [unwired: 1 in, 1 out]
      n170 = call <userlib>:"Remove.vi"("Module ID"=w493, "CloneRegRef"=w494) -> ("error out"=w499:errorcluster)  [unwired: 7 in, 2 out]
      n171 = flat-sequence {
        tunnel: w500 -> [w503]
        tunnel: w499 -> [_]
        tunnel: [w501] -> w498
        frame #0 {
          w502 = T11 2 items=["no dialog", "OK message", "continue or stop message", "OK message + warnings", "continue/stop + warnings"] ("type of dialog (OK msg:1)")
          n172 = call <vilib>:"Simple Error Handler.vi"("type of dialog (OK msg:1)"=w502, "error in (no error)"=w503) -> ("error out"=w501:errorcluster)  [unwired: 3 in, 4 out]
        }
      }
    }
  }
  n173 = call "DestroyClone.vi"("error in (no error)"=w7, "Exit via Stop Module Req?"=w3, "Wait for Module to stop?"=w4, "ModuleAdmin"=w5) -> ("error out"=w6:errorcluster, "External Launch"=w2:bool)  [unwired: 5 in, 1 out]
  n174 = Release Queue(queue=w12, error in (no error)=w6) -> (error out=w1:errorcluster)  [unwired: 1 in, 2 out]
  "error out" <- w1
  n175 = case shown="True" w2 {
    tunnel: w1 -> [_ w505]
    frame False {
    }
    frame True {
      n176 = control-ref of="This VI"() -> (w504:refnum<vi>)
      n177 = case shown="Error" w505 {
        tunnel: w504 -> [w506 w507]
        frame No Error {
          n178 = invoke class="VI" method="FP.Close"(reference=w506) -> ()  [unwired: 2 in, 3 out]
        }
        frame Error {
          n179 = invoke class="VI" method="FP.Open"(reference=w507, "Activate"=TRUE ("Activate?")) -> ()  [unwired: 3 in, 5 out]
        }
      }
    }
  }
